vi "SVT Running RMS Level (N Ch).vi"(6 "restart averaging (F)":bool, 8 "error in (no error)":errorcluster, 9 "integration time [s]":dbl=1.0 format="%.2f", 11 "scaled signals [EU]":waveform(dbl)[](array[waveform])) -> (0 "error out":errorcluster, 1 "actual integration time [s]":dbl=nan format="%.2f", 2 "unit labels":string[](array[string]), 3 "running RMS levels [EU rms]":dbl[](array[numeric])=[nan] format="%.2f")   [LabVIEW 2017]
doc: "Computes the running root-mean-square (RMS) level of <B>scaled signal [EU]</B> or <B>even angle signal [EU]</B>. <B>integration time [s]</B> and <B>integration revolutions</B> specify the duration over which the RMS level is computed. You can use this polymorphic VI to compute the running RMS level for a single channel or for N channels, or for a single channel or N channels of resampled data. The data type you wire to the <B>scaled signal [EU]</B> or <B>even angle signal [EU]</B> input determines the polymorphic instance to use."
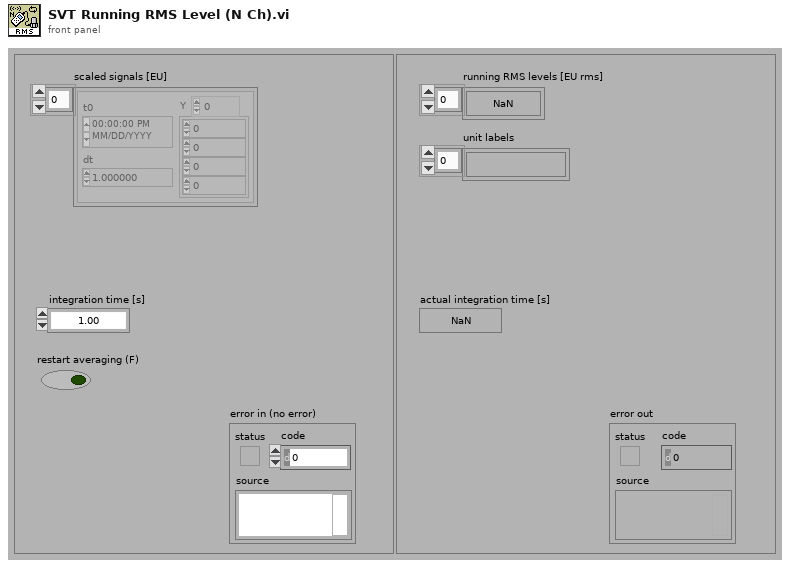
[diagram p1: front panel]
types:
  T1 = enum16{"RMS", "Running RMS", "Exp avg  ", "Dec exp avg ", "Peak", "Crest"}
  T2 = enum16{"Reset filter", "Restart averaging", "Continue processing"}
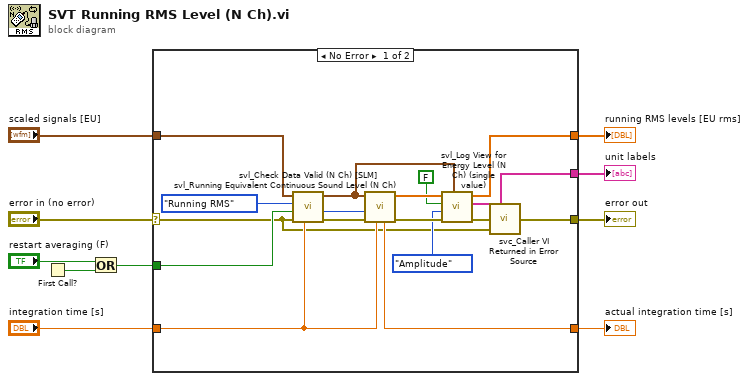
[diagram p0: block diagram]
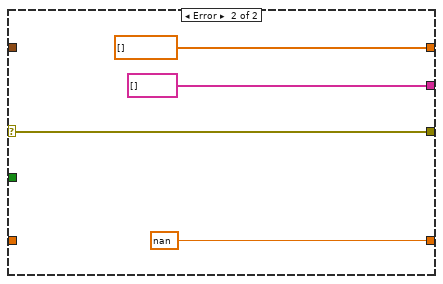
[diagram p2: hidden frame]
diagram:
  n1 = First Call?() -> (First Call?: T/F=w4:bool)
  n2 = Or(x="restart averaging (F)", y=w4) -> (x .or. y?=w2:bool)
  n3 = case shown="No Error" "error in (no error)" {
    selector: "error in (no error)" -> [w11 w31]
    tunnel: [w20 w31] -> w10
    tunnel: [w19 nan ("actual integration time [s]")] -> w9
    tunnel: [w24 dbl[] [] ("energy levels [EU^2 rms]")] -> w8
    tunnel: [w23 string[] [] ("unit label [ ]")] -> w7
    tunnel: "integration time [s]" -> [w15 _]
    tunnel: "scaled signals [EU]" -> [w13 _]
    tunnel: w2 -> [w17 _]
    frame No Error {
      n4 = call <vilib>:"svl_Check Data Valid (N Ch) [SLM].vi"("integration time [s]"=w15, "error in (no error)"=w11, "restart averaging (F)"=w17, "level analysis"=T1."Running RMS" ("Level Analysis"), "scaled signals [EU]"=w13) -> ("error out"=w18:errorcluster, "processing state"=w16:T2, "dup scaled signals [EU]"=w12:waveform(dbl)[])  [unwired: 4 in]
      n5 = call <vilib>:"svl_Running Equivalent Continuous Sound Level (N Ch).vi"("integration time [s]"=w15, "error in (no error)"=w18, "processing state"=w16, "scaled signals [EU]"=w12) -> ("error out"=w26:errorcluster, "energy level [ ] [EU^2 rms]"=w27:dbl[], "actual integration time [s]"=w19:dbl)  [unwired: 5 in]
      n6 = call <vilib>:"svl_Log View for Energy Level (N Ch) (single value).vi"("waveform parameters"=w12, "error in (no error)"=w26, "view mode"=enum16{"Power", "Amplitude"}."Amplitude", "dB On (T)"=FALSE, "energy levels [EU^2 rms]"=w27) -> ("error out"=w25:errorcluster, "unit label [ ]"=w23:string[], "energy levels [EU^2 rms]"=w24:dbl[])  [unwired: 4 in]
      n7 = call <vilib>:"svc_Caller VI Returned in Error Source.vi"("warning input to caller"=w11, "error in (no error)"=w25) -> ("error out"=w20:errorcluster)  [unwired: 3 in]
    }
    frame Error {
    }
  }
  "running RMS levels [EU rms]" <- w8
  "unit labels" <- w7
  "actual integration time [s]" <- w9
  "error out" <- w10
